vi "Run.vi"(8 "error in (no error)":errorcluster caption="entrée d'erreur (pas d'erreur)", 11 "Classification.lvclass":refnum<class "Classification.lvclass">) -> (0 "error out":errorcluster caption="sortie d'erreur", 2 "Data":T1, 3 "Classification.lvclass":refnum<class "Classification.lvclass">)   [LabVIEW 2020, in "Classification.lvclass"]
doc: "Returns : \n\nX : array of shape [n_samples, n_features]\n The generated samples.\n\ny : array of shape [n_samples]\n The integer labels for class membership of each sample."
uses:
  Classification.lvclass
  Classification.lvclass/Classification.ctl
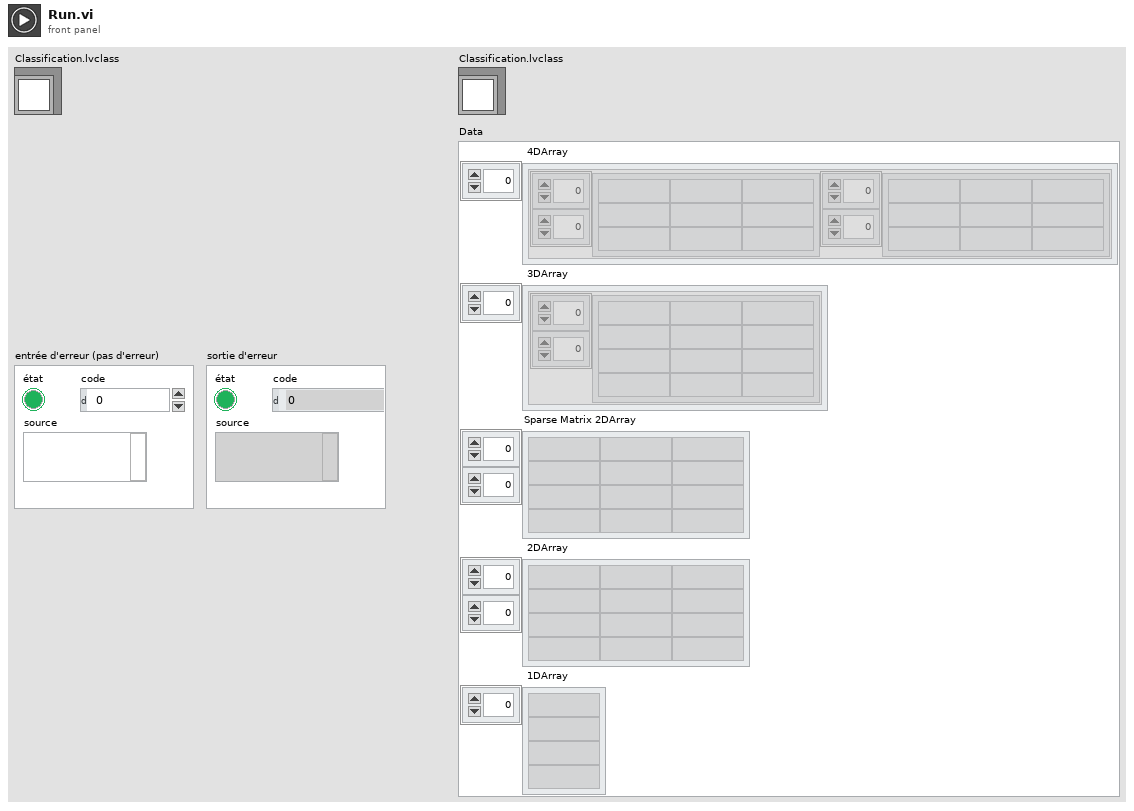
[diagram p1: front panel]
types:
  T1 = cluster{" 4DArray":cluster{"1":string[][], "2":string[][]}[], " 3DArray":cluster{"Tableau":string[][]}[], "Sparse Matrix 2DArray":string[][], " 2DArray":string[][], " 1DArray":string[]}
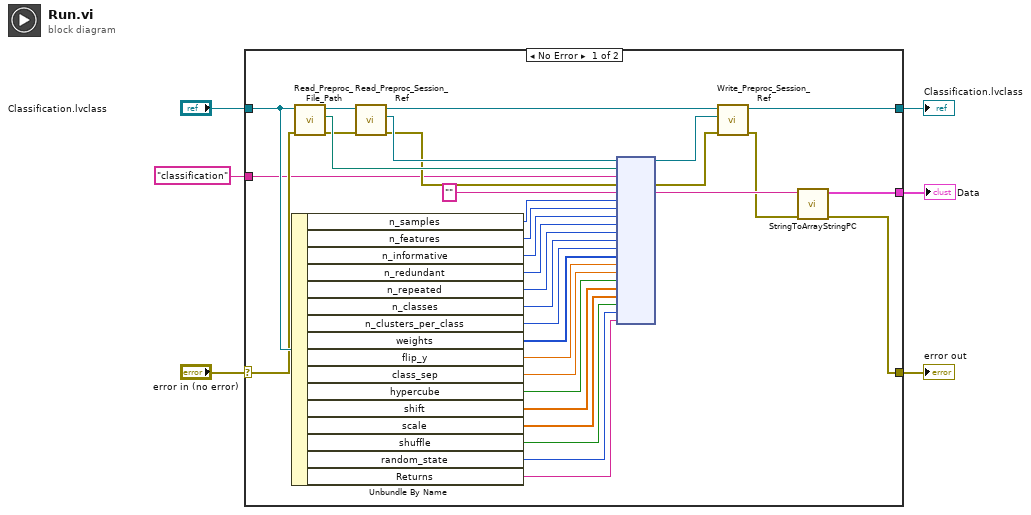
[diagram p0: block diagram]
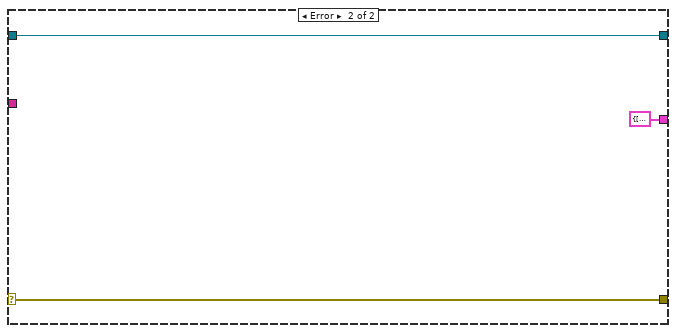
[diagram p2: hidden frame]
diagram:
  n1 = case shown="No Error" "error in (no error)" {
    selector: "error in (no error)" -> [w21 w42]
    tunnel: [w8 w42] -> w5
    tunnel: [w11 w41] -> w3
    tunnel: "Classification.lvclass" -> [w22 w41]
    tunnel: "classification" -> [w20 _]
    tunnel: [w7 T1 {" 4DArray"=[], " 3DArray"=[], "Sparse Matrix 2DArray"=[], " 2DArray"=[], " 1DArray"=[]} ("Data")] -> w1
    frame No Error {
      n2 = Unbundle By Name(w22) -> ("n_samples"=w30:u32, "n_features"=w29:u32, "n_informative"=w28:i32, "n_redundant"=w27:i32, "n_repeated"=w26:i32, "n_classes"=w25:u32, "n_clusters_per_class"=w24:u32, "weights"=w23:i32[], "flip_y"=w19:dbl, "class_sep"=w18:dbl, "hypercube"=w17:bool, "shift"=w16:dbl[], "scale"=w15:dbl[], "shuffle"=w14:bool, "random_state"=w13:i32, "Returns"=w12:string)
      n3 = call-dynamic "Read_Preproc_File_Path.vi"("error in (no error)"=w21, "Python in"=w22) -> ("error out"=w34:errorcluster, "File_Path"=w37:path, "Python out"=w39:refnum<class "Classification.lvclass">)  [unwired: 7 in]
      n4 = call-dynamic "Read_Preproc_Session_Ref.vi"("error in (no error)"=w34, "Python in"=w39) -> ("error out"=w35:errorcluster, "Session_ref"=w36:refnum<k35>, "Python out"=w38:refnum<class "Classification.lvclass">)  [unwired: 7 in]
      n5 = node(w36, w37, w20, w35, "", w30, w29, w28, w27, w26, w25, w24, w23, w19, w18, w17, w16, w15, w14, w13, w12) -> (w31:refnum<k35>, w33:errorcluster, w10:string)  [unwired: 16 in, 2 out]
      n6 = call-dynamic "Write_Preproc_Session_Ref.vi"("error in (no error)"=w33, "Session_ref"=w31, "Python in"=w38) -> ("error out"=w9:errorcluster, "Python out"=w11:refnum<class "Classification.lvclass">)  [unwired: 7 in]
      n7 = call "StringToArrayStringPC.vi"("sortie d'erreur"=w9, "Return value"=w10) -> ("sortie d'erreur"=w8:errorcluster, "Data"=w7:T1)  [unwired: 8 in]
    }
    frame Error {
    }
  }
  "error out" <- w5
  "Classification.lvclass" <- w3
  "Data" <- w1
